vi "poll_and_write_LiCor_data.vi"(8 "file error in":errorcluster, 9 "file ref in":refnum<file>, 10 "LiCor error in":errorcluster, 11 "LiCor session in":refnum<visa-resource-name>="COM1") -> (0 "file error out":errorcluster, 1 "file ref out":refnum<file>, 2 "LiCor error out":errorcluster, 3 "LiCor session out":refnum<visa-resource-name>="COM1", 4 "pCO2":dbl)   [LabVIEW 2010]
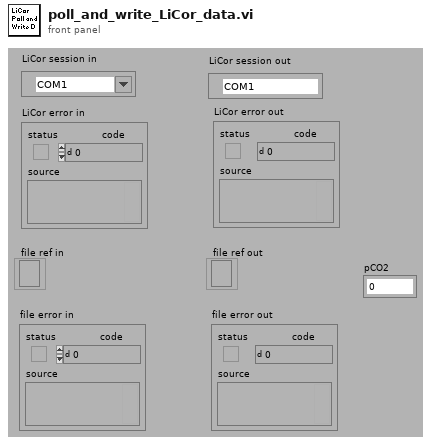
[diagram p1: front panel]
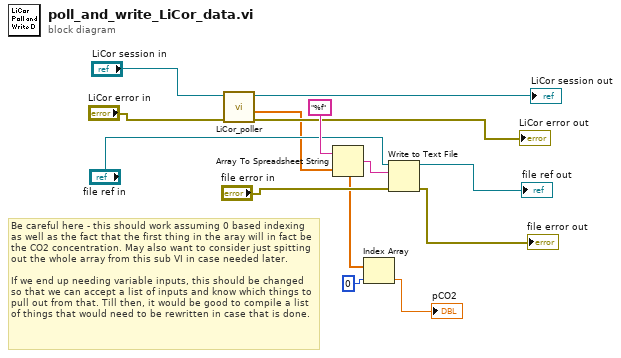
[diagram p0: block diagram]
diagram:
  # "Be careful here - this should work assuming 0 based indexing as well as the fact that the first thing in the aray will in fact be the CO2 concentration. May also want to consider just spitting out the whole array from this sub VI in case needed later. \n\nIf we end up needing variable inputs, this should be changed so that we can accept a list of inputs and know which things to pull out from that. Till then, it would be good to compile a list of things that would need to be rewritten in case that is done."
  n1 = call "LiCor_poller.vi"("error in"="LiCor error in", "VISA session in"="LiCor session in") -> ("error out"=→"LiCor error out":errorcluster, "data array"=w3:dbl[], "VISA session out"=→"LiCor session out":refnum<visa-resource-name>)  [unwired: 5 in, 2 out]
  n2 = Array To Spreadsheet String(array=w3, 3:"%f") -> (spreadsheet string=w13:string)  [unwired: 1 in]
  n3 = Index Array(array=w3, index=0) -> (element=→"pCO2":dbl)
  n4 = Write to Text File(file (use dialog)="file ref in", text=w13, error in="file error in") -> (refnum out=→"file ref out":refnum<file>, error out=→"file error out":errorcluster)  [unwired: 1 in, 1 out]
